vi "Display Elements Test Panel.vi"() -> ()   [LabVIEW 2021]
uses:
  Graph/Public/Controls/Fill To.ctl
  Graph/Public/Controls/Range.ctl
  Display Utilities/Public/Controls/2D Dimensions.ctl
  Display Utilities/Public/Controls/2D Coordinates.ctl
  Pixel/Pixel.lvclass
  C:/Git/MEMOSFET/myRIO-Neopixel/Source/RT/Display Element/Display Element.lvclass
  Square/Square.lvclass
  String/String.lvclass
  Graph/Graph.lvclass
  Display Element/Display Element.lvclass
  Display/Display Manager.lvclass
  Display Utilities/Display Utilities.lvlib
panel:
  in  "Display X":i32=24 caption="X"
  in  "Display Y":i32=8 caption="Y"
  in  "Position X":i32 caption="X"
  in  "Position Y":i32 caption="Y"
  in  "Force X":i32 caption="X"
  in  "Force Y":i32 caption="Y"
  in  "Tag":string
  in  "Layer":u32
  in  "Delete If Outside Bounds":bool=TRUE
  in  "Color":u32(colorbox)
  in  "Create Button":bool
  in  "Element Type":enum32{"Pixel", "Square", "String", "Graph"}(tab)
  in  "Trace":i32
  in  "Height":u32
  in  "Width":u32
  in  "Text":string
  in  "Width G":u32 caption="Width"
  in  "Height G":u32 caption="Height"
  in  "Data":i32[](array[numeric])
  in  "Fill To":T1
  in  "Range":T2
  out "Frame":u32[][](array[colorbox])
  in  "stop":bool
  # "Display Settings"
  # "Display Size"
  # "Display Elements Creation"
  # "Position"
  # "Force"
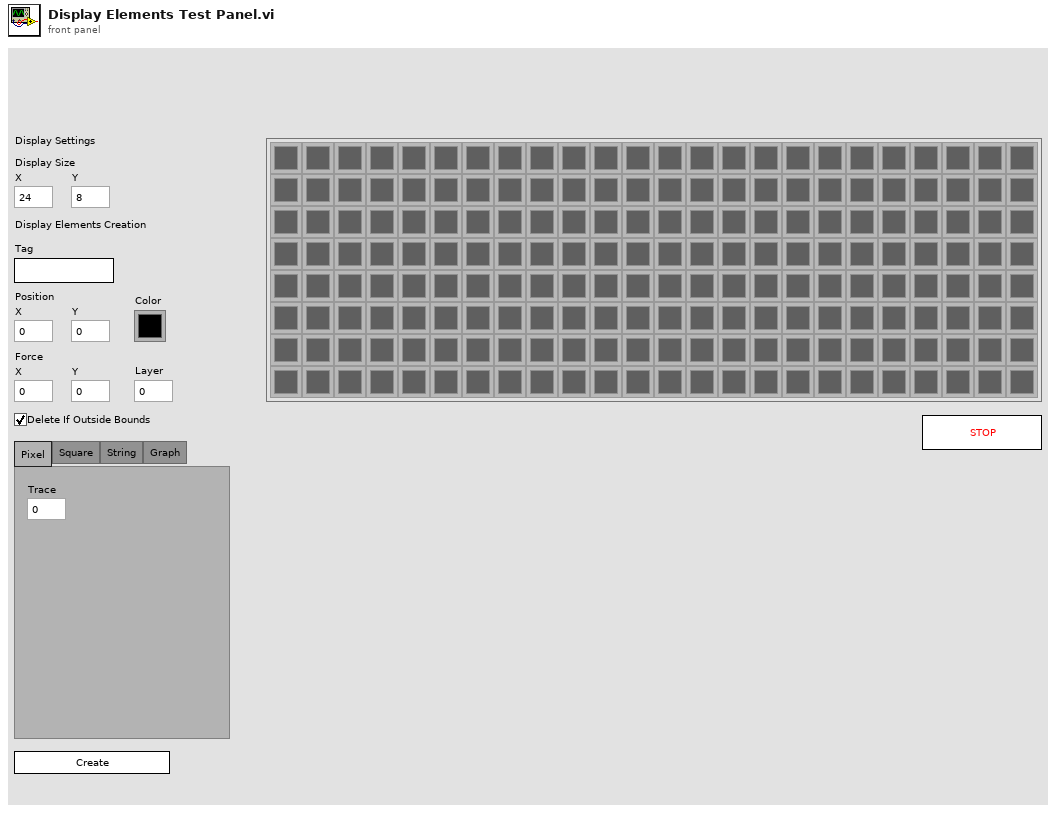
[diagram p1: front panel]
types:
  T1 = typedef "Graph.lvclass/Fill To.ctl" = enum16{"None", "Inf", "-Inf"}
  T2 = typedef "Graph.lvclass/Range.ctl" = cluster{"Maximum":dbl, "Minimum":dbl}
  T3 = typedef "Display Utilities.lvlib/2D Dimensions.ctl" = cluster{"Width":i32, "Height":i32}
  T4 = typedef "Display Utilities.lvlib/2D Coordinates.ctl" = cluster{"X":i32, "Y":i32}
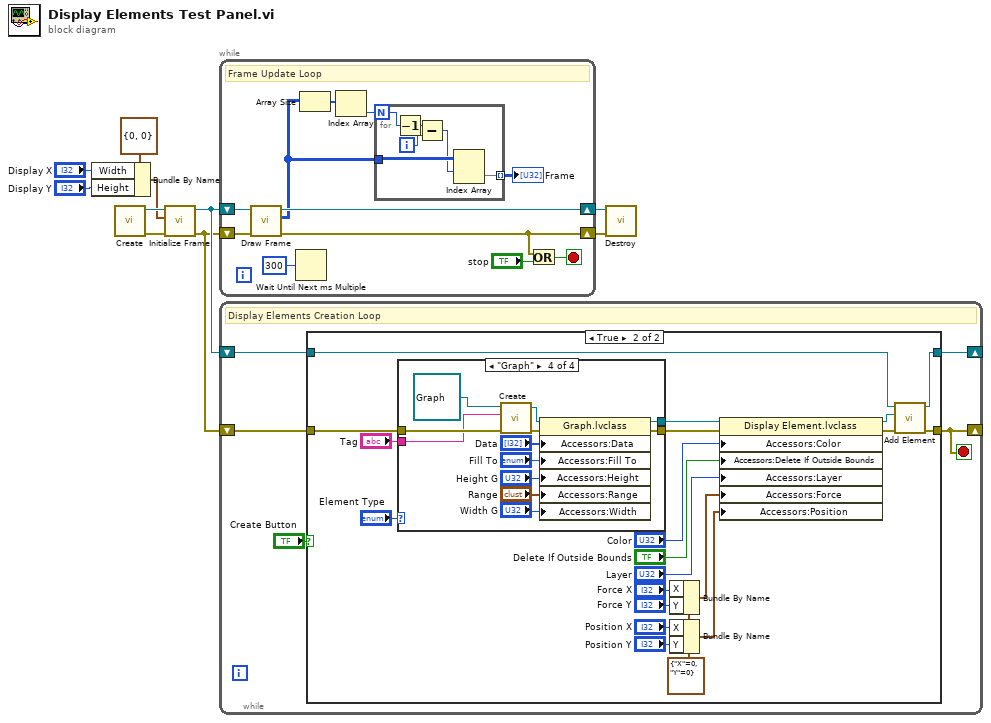
[diagram p0: block diagram]
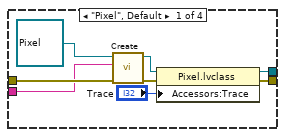
[diagram p3: hidden frame]
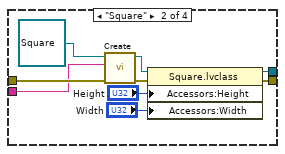
[diagram p4: hidden frame]
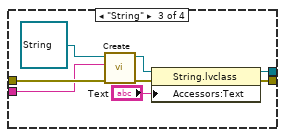
[diagram p5: hidden frame]
diagram:
  n1 = Bundle By Name(cluster=T3 {"Width"=0, "Height"=0} ("Size"), "Width"="Display X", "Height"="Display Y") -> (w1:T3)
  n2 = call "Create.vi"() -> ("Error Out"=w7:errorcluster, "Screen Out"=w8:refnum<class "Display Manager.lvclass">)  [unwired: 10 in]
  n3 = call "Initialize Frame.vi"("Error In"=w7, "Size"=w1, "Display In"=w8) -> ("Error Out"=w5:errorcluster, "Display Out"=w6:refnum<class "Display Manager.lvclass">)  [unwired: 7 in]
  n4 = while {
    shift-right: [w19] -> w9
    shift-left: w5 -> [w14]
    shift-right: [w21] -> w10
    shift-left: w6 -> [w13]
    stop <- w17 stop-if-true
    # "Frame Update Loop"
    n5 = call "Draw Frame.vi"("Error In"=w14, "Display In"=w13) -> ("Error Out"=w19:errorcluster, "Frame"=w11:u32[][], "Display Out"=w21:refnum<class "Display Manager.lvclass">)  [unwired: 7 in]
    n6 = Wait Until Next ms Multiple(millisecond multiple=u32 300) -> ()  [unwired: 1 out]
    n7 = Array Size(array=w11) -> (size(s)=w16:i32[])
    n8 = Index Array(array=w16) -> (element=w15:i32)  [unwired: 1 in]
    n9 = for {
      N: w15 -> [w24]
      tunnel: w11 -> [w26]
      tunnel: [w22] -> w12 mode=indexing
      i -> [w27]
      n10 = Decrement(x=w24) -> (x-1=w23:i32)
      n11 = Subtract(x=w23, y=w27) -> (x-y=w25:i32)
      n12 = Index Array(array=w26, index (row)=w25) -> (element=w22:u32[])  [unwired: 1 in]
    }
    "Frame" <- w12
    n13 = Or(x=w19, y="stop") -> (x .or. y?=w17:bool)
  }
  n14 = while {
    shift-right: [w30] -> _
    shift-left: w6 -> [w32]
    shift-right: [w29] -> _
    shift-left: w5 -> [w31]
    stop <- w29 stop-if-true
    # "Display Elements Creation Loop"
    n15 = case shown="True" "Create Button" {
      tunnel: w32 -> [w33 w54]
      tunnel: w31 -> [w34 w50]
      tunnel: [w33 w53] -> w30
      tunnel: [w34 w52] -> w29
      frame False {
      }
      frame True {
        w42 = T4 {"X"=0, "Y"=0} ("Force")
        n16 = case shown="\"Graph\"" "Element Type" {
          tunnel: w50 -> [w62 w71 w79 w83]
          tunnel: [w57 w66 w74 w90] -> w49
          tunnel: [w58 w65 w75 w91] -> w48
          tunnel: "Tag" -> [w56 w64 w73 w82]
          frame "Pixel", Default {
            n17 = call-dynamic "Create.vi"("Error In"=w62, "Tag"=w56, "Pixel In"=refnum<class "Pixel.lvclass"> refnum ("Pixel.lvclass")) -> ("Error Out"=w60:errorcluster, "Pixel Out"=w61:refnum<class "Pixel.lvclass">)  [unwired: 7 in]
            n18 = property class="Pixel.lvclass"(reference=w61, error in=w60, "Accessors:Trace"="Trace") -> (reference out=w58:refnum<class "Pixel.lvclass">, error out=w57:errorcluster)
          }
          frame "Square" {
            n19 = call-dynamic "Create.vi"("Error In"=w71, "Tag"=w64, "Square In"=refnum<class "Square.lvclass"> refnum ("Square.lvclass")) -> ("Error Out"=w69:errorcluster, "Square Out"=w70:refnum<class "Square.lvclass">)  [unwired: 7 in]
            n20 = property class="Square.lvclass"(reference=w70, error in=w69, "Accessors:Height"="Height", "Accessors:Width"="Width") -> (reference out=w65:refnum<class "Square.lvclass">, error out=w66:errorcluster)
          }
          frame "String" {
            n21 = call-dynamic "Create.vi"("Error In"=w79, "Tag"=w73, "Pixel In"=refnum<class "String.lvclass"> refnum ("String.lvclass")) -> ("Error Out"=w77:errorcluster, "Pixel Out"=w78:refnum<class "String.lvclass">)  [unwired: 7 in]
            n22 = property class="String.lvclass"(reference=w78, error in=w77, "Accessors:Text"="Text") -> (reference out=w75:refnum<class "String.lvclass">, error out=w74:errorcluster)
          }
          frame "Graph" {
            n23 = call-dynamic "Create.vi"("Error In"=w83, "Tag"=w82, "Graph In"=refnum<class "Graph.lvclass"> refnum ("Graph.lvclass")) -> ("Error Out"=w81:errorcluster, "Graph Out"=w80:refnum<class "Graph.lvclass">)  [unwired: 7 in]
            n24 = property class="Graph.lvclass"(reference=w80, error in=w81, "Accessors:Data"="Data", "Accessors:Fill To"="Fill To", "Accessors:Height"="Height G", "Accessors:Range"="Range", "Accessors:Width"="Width G") -> (reference out=w91:refnum<class "Graph.lvclass">, error out=w90:errorcluster)
          }
        }
        n25 = Bundle By Name(cluster=w42, "X"="Force X", "Y"="Force Y") -> (w41:T4)
        n26 = Bundle By Name(cluster=w42, "X"="Position X", "Y"="Position Y") -> (w40:T4)
        n27 = property class="Display Element.lvclass"(reference=w48, error in=w49, "Accessors:Color"="Color", "Accessors:Delete If Outside Bounds"="Delete If Outside Bounds", "Accessors:Layer"="Layer", "Accessors:Force"=w41, "Accessors:Position"=w40) -> (reference out=w46:refnum<class "Display Element.lvclass">, error out=w45:errorcluster)
        n28 = call "Add Element.vi"("Error In"=w45, "New Element"=w46, "Display In"=w54) -> ("Error Out"=w52:errorcluster, "Display Out"=w53:refnum<class "Display Manager.lvclass">)  [unwired: 7 in]
      }
    }
  }
  n29 = call "Destroy.vi"("Error In"=w9, "Display In"=w10) -> ()  [unwired: 9 in, 1 out]
